vi "CalculatorExpressionTest.vi"() -> ()   [LabVIEW 2019]
uses:
  Library/Eval.lvlib
panel:
  out "Array":cluster{string, bool}[](array[cluster])
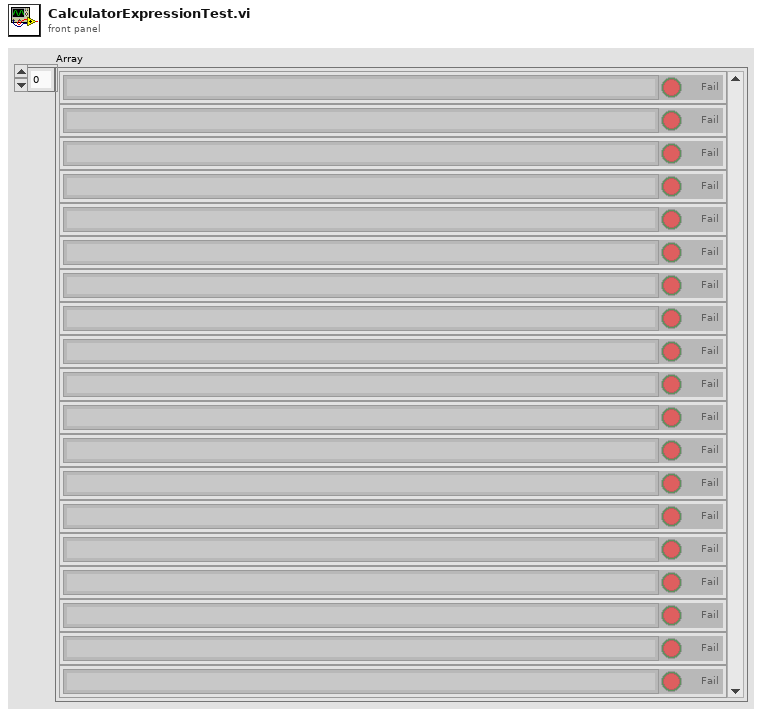
[diagram p1: front panel]
types:
  T1 = cluster{"String":string, cluster{"Start":i32, "End":i32, "Token":enum16{"ADD", "BITAND", "BITOR", "COMMA", "DIV", "Dnumeric", "EQUAL", "EXP", "FUNC", "GREATER", "GREATEREQ", "INumeric", "Identifier", "Ignore", "LESS", "LESSEQ", "LOGAND", "LOGOR", "LPAR", "LSHIFT", "MULT", "N/A", "RPAR", "RSHIFT", "SUB", "UADD", "USUB"}}[]}
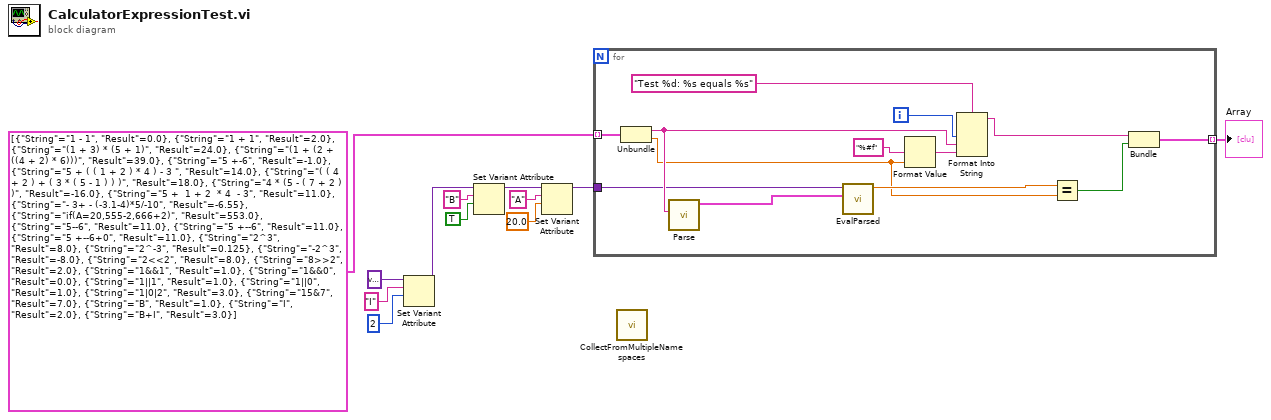
[diagram p0: block diagram]
diagram:
  n1 = Set Variant Attribute(Variant=variant ("variant"), name="I", value=2) -> (Variant out=w1:variant)  [unwired: 1 in, 2 out]
  n2 = Set Variant Attribute(Variant=w1, name="B", value=TRUE) -> (Variant out=w7:variant)  [unwired: 1 in, 2 out]
  n3 = Set Variant Attribute(Variant=w7, name="A", value=20.0 ("element")) -> (Variant out=w9:variant)  [unwired: 1 in, 2 out]
  n4 = for {
    tunnel: cluster{"String":string, "Result":dbl}[] [{"String"="1 - 1", "Result"=0.0}, {"String"="1 + 1", "Result"=2.0}, {"String"="(1 + 3) * (5 + 1)", "Result"=24.0}, {"String"="(1 + (2 + ((4 + 2) * 6)))", "Result"=39.0}, {"String"="5 +-6", "Result"=-1.0}, {"String"="5 + ( ( 1 + 2 ) * 4 ) - 3 ", "Result"=14.0}, {"String"="( ( 4 + 2 ) + ( 3 * ( 5 - 1 ) ) )", "Result"=18.0}, {"String"="4 * (5 - ( 7 + 2 ) )", "Result"=-16.0}, {"String"="5 +  1 + 2  * 4  - 3", "Result"=11.0}, {"String"="- 3+ - (-3.1-4)*5/-10", "Result"=-6.55}, {"String"="if(A=20,555-2,666+2)", "Result"=553.0}, {"String"="5--6", "Result"=11.0}, {"String"="5 +--6", "Result"=11.0}, {"String"="5 +--6+0", "Result"=11.0}, {"String"="2^3", "Result"=8.0}, {"String"="2^-3", "Result"=0.125}, {"String"="-2^3", "Result"=-8.0}, {"String"="2<<2", "Result"=8.0}, {"String"="8>>2", "Result"=2.0}, {"String"="1&&1", "Result"=1.0}, {"String"="1&&0", "Result"=0.0}, {"String"="1||1", "Result"=1.0}, {"String"="1||0", "Result"=1.0}, {"String"="1|0|2", "Result"=3.0}, {"String"="15&7", "Result"=7.0}, {"String"="B", "Result"=1.0}, {"String"="I", "Result"=2.0}, {"String"="B+I", "Result"=3.0}] -> [w25] mode=indexing
    tunnel: w9 -> [w18]
    tunnel: [w13] -> w2 mode=indexing
    i -> [w21]
    n5 = Unbundle(w25) -> ("String"=w20:string, "Result"=w16:dbl)
    n6 = call "Parse.vi"("String"=w20) -> ("ParsedExpression"=w19:T1)  [unwired: 9 in, 1 out]
    n7 = call "EvalParsed.vi"("Cluster"=w19, "NameSpace"=w18) -> ("element"=w17:dbl)  [unwired: 9 in]
    n8 = Format Value(format string="%#f", value (0)=w16) -> (output string=w22:string)  [unwired: 1 in]
    n9 = Format Into String(format string="Test %d: %s equals %s", w21, w20, w22) -> (resulting string=w15:string)  [unwired: 2 in, 1 out]
    n10 = Equal?(x=w17, y=w16) -> (x = y?=w14:bool)
    n11 = Bundle(w15, w14) -> (w13:cluster{string, bool})  [unwired: 1 in]
  }
  "Array" <- w2
  n12 = call "CollectFromMultipleNamespaces.vi"() -> ()  [unwired: 11 in, 1 out]
